vi "Write Communicator.vi"(8 "error in (no error)":errorcluster, 10 "Communicator.lvclass":refnum<class "Communicator.lvclass">, 11 "CoolerControler in":refnum<class "CoolerControler.lvclass">) -> (0 "error out":errorcluster, 3 "CoolerControler out":refnum<class "CoolerControler.lvclass">)   [LabVIEW 2016, in "CoolerControler.lvclass"]
uses:
  CoolerControler.lvclass
  common_serial_tcpextended/Communicator/Communicator.lvclass
  CoolerControler.lvclass/CoolerControler.ctl
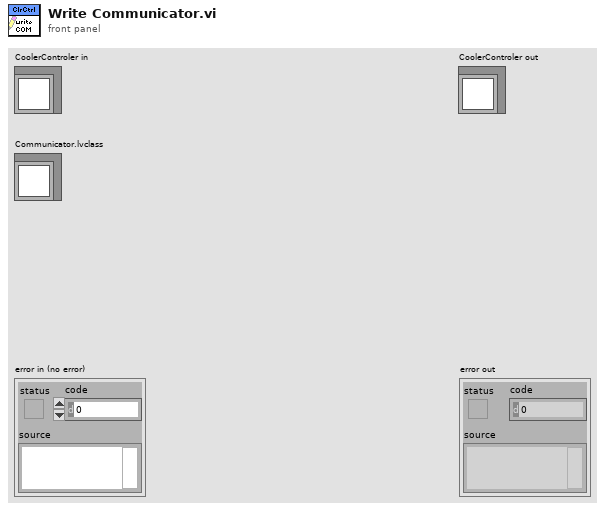
[diagram p1: front panel]
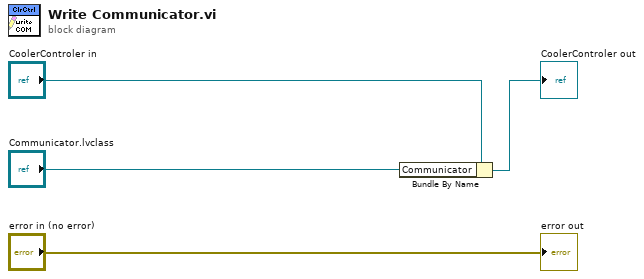
[diagram p0: block diagram]
diagram:
  n1 = Bundle By Name(cluster="CoolerControler in", "Communicator"="Communicator.lvclass") -> (→"CoolerControler out":refnum<class "CoolerControler.lvclass">)
  "error out" <- "error in (no error)"
